vi "AddTAFMenu.vi"(8 "ErrorIn":errorcluster, 10 "MenuIn":T1[](array[typedef]), 11 "MasterGUIIn":refnum<class "MasterGUI.lvclass">) -> (0 "ErrorOut":errorcluster, 2 "MenuOut":T1[](array[typedef]), 3 "MasterGUIOut":refnum<class "MasterGUI.lvclass">)   [LabVIEW 2021, in "MasterGUI.lvclass"]
uses:
  MasterGUI.lvclass
  MenuItem.ctl
  MasterGUI.lvclass/MasterGUI.ctl
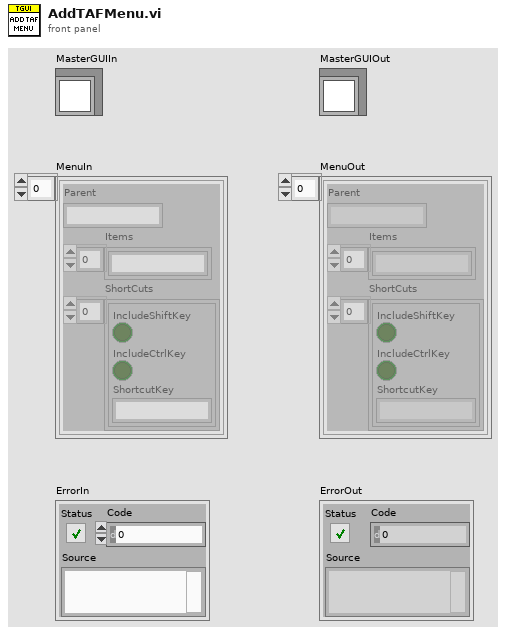
[diagram p1: front panel]
types:
  T1 = typedef "MasterGUI.lvclass/MenuItem.ctl" = cluster{"Parent":string, "Items":string[], "ShortCuts":cluster{"IncludeShiftKey":bool, "IncludeCtrlKey":bool, "ShortcutKey":string}[]}
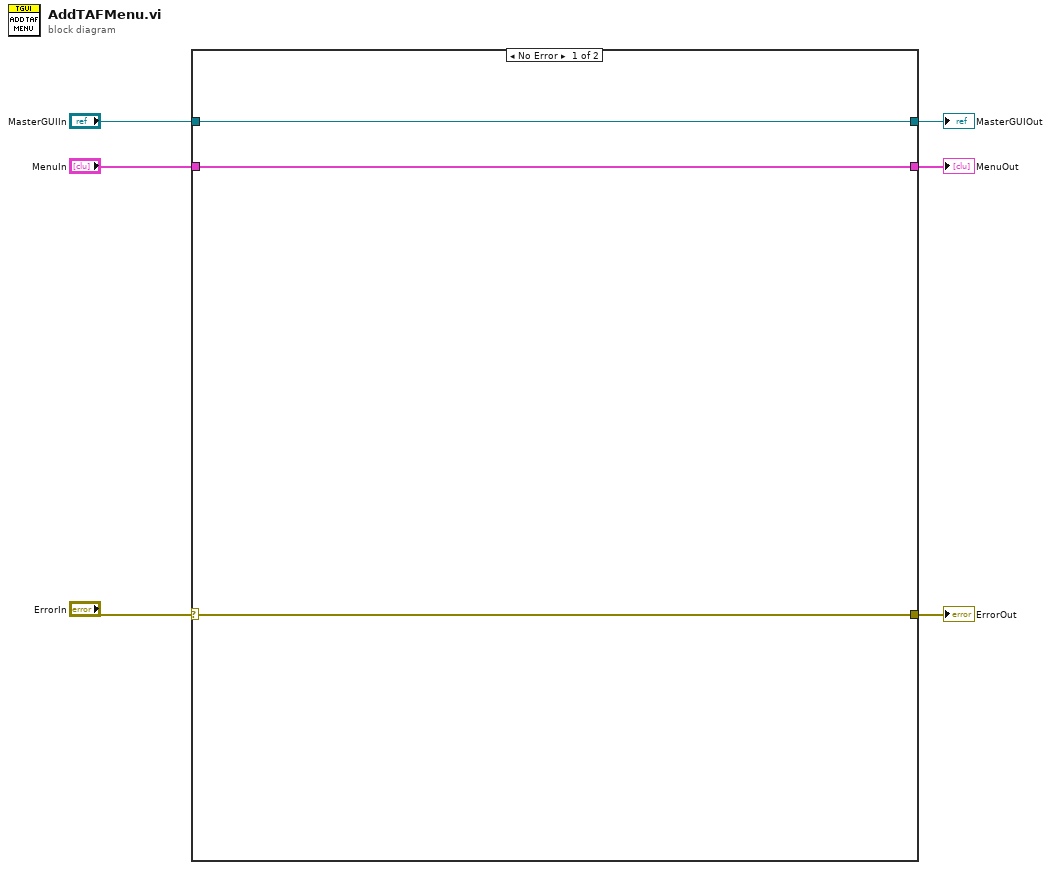
[diagram p0: block diagram]
diagram:
  n1 = case shown="No Error" "ErrorIn" {
    selector: "ErrorIn" -> [w9 w12]
    tunnel: [w9 w12] -> w6
    tunnel: [w8 w10] -> w4
    tunnel: [w7 w11] -> w2
    tunnel: "MasterGUIIn" -> [w7 w11]
    tunnel: "MenuIn" -> [w8 w10]
    frame No Error {
    }
    frame Error {
    }
  }
  "MasterGUIOut" <- w2
  "ErrorOut" <- w6
  "MenuOut" <- w4
